vi "SwerveGlobals.vi"() -> ()   [LabVIEW 2017]
panel:
  in  "GyroOffset":dbl
  in  "Gyro":dbl
  in  "SwerveOffsets":dbl[](array[numeric])
  in  "ZAxis":dbl
  in  "YAxis":dbl
  in  "XAxis":dbl
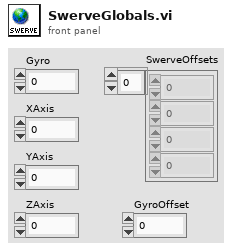
[diagram p1: front panel]
diagram:
